vi "DiffDriveTrainSim_ToughBoxMiniGearRatio.vi"(11 "ToughBoxMiniGear":T1) -> (3 "GearRatio":dbl)   [LabVIEW 2019, in "Trajectory_Library.lvlib"]
doc: "Convience function to allow user to select kit bot gear ratio from an enum selector and return the ratio value\n\nInput:\n - StandardGearRatios -- Enumerated gear ratio selector\n\nOutput:\n - GearRatio -- Gear ratio value."
uses:
  Trajectory_Library.lvlib
  Enum/DIFF_DRIVE_ToughBoxMini_GearChoice_ENUM.ctl
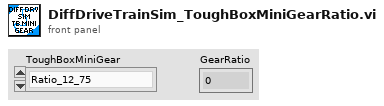
[diagram p1: front panel]
types:
  T1 = typedef "Trajectory_Library.lvlib/DIFF_DRIVE_ToughBoxMini_GearChoice_ENUM.ctl" = enum16{"Ratio_12_75", "Ratio_10_71", "Ratio_8_45", "Ratio_7_31", "Ratio_5_95"}
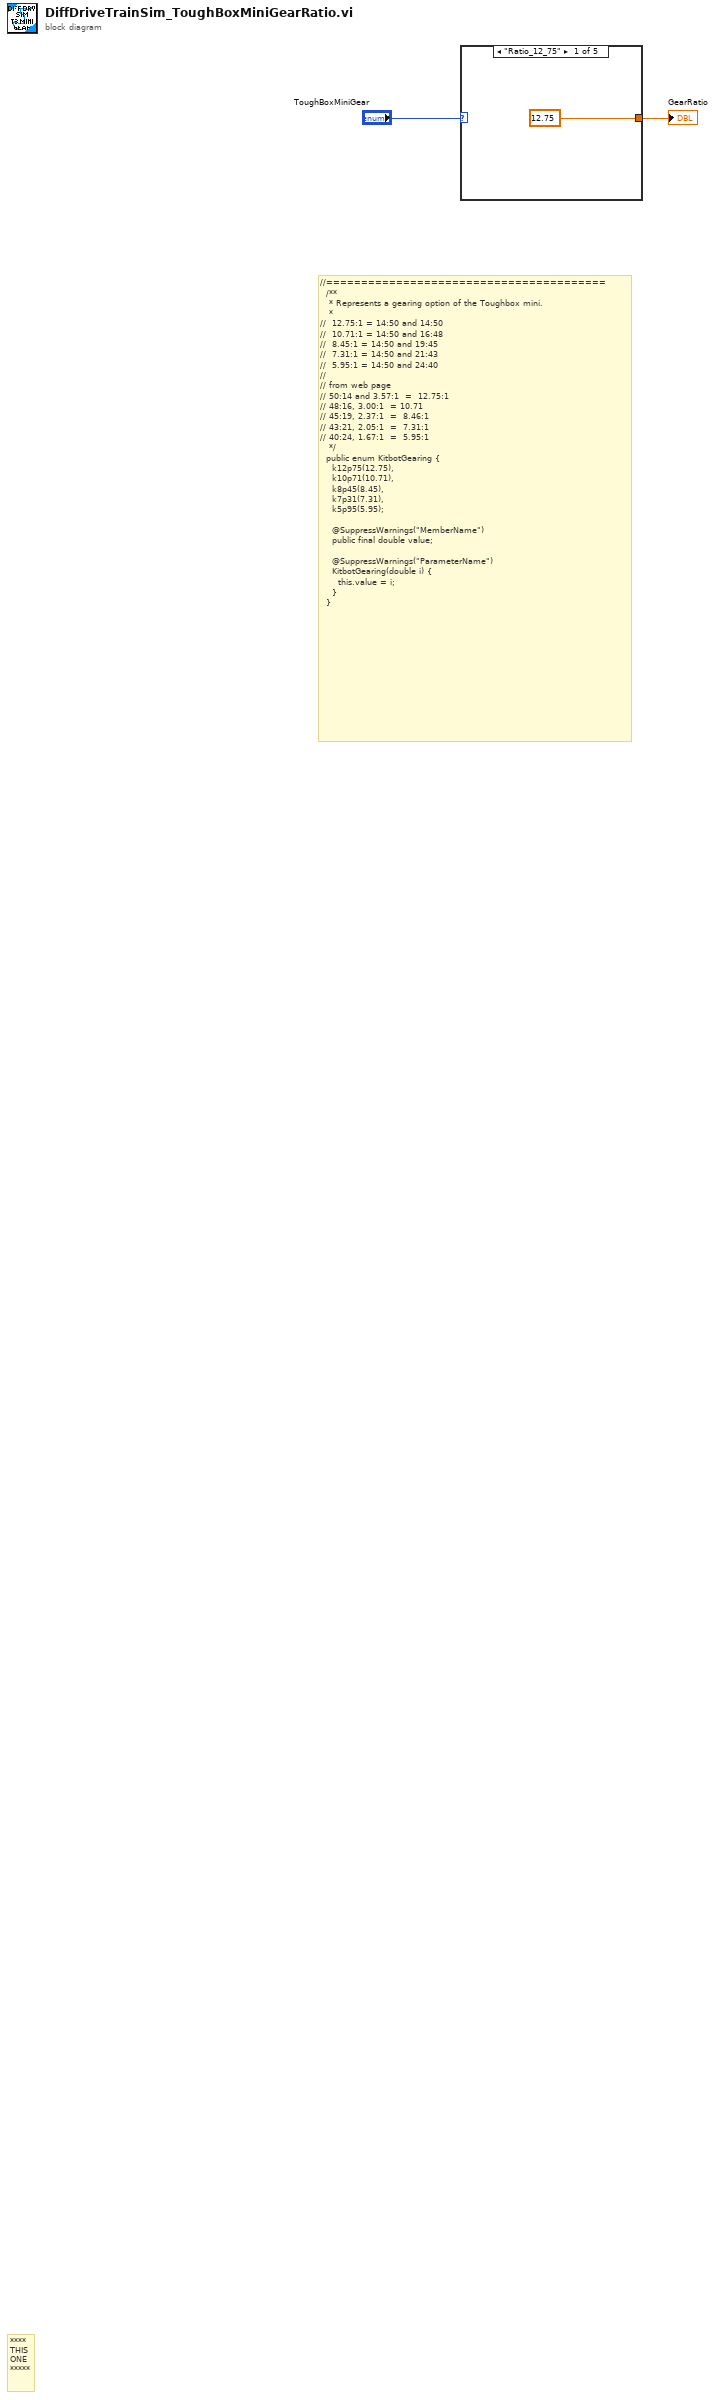
[diagram p0: block diagram]
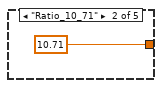
[diagram p2: hidden frame]
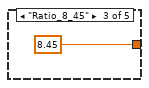
[diagram p3: hidden frame]
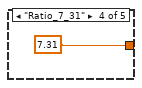
[diagram p4: hidden frame]
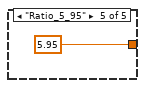
[diagram p5: hidden frame]
diagram:
  # "//========================================\n  /**\n   * Represents a gearing option of the Toughbox mini. \n   *\n//\t\t12.75:1 = 14:50 and 14:50 \n//\t\t10.71:1 = 14:50 and 16:48 \n//\t\t8.45:1 = 14:50 and 19:45\n//\t\t7.31:1 = 14:50 and 21:43\n//\t\t5.95:1 = 14:50 and 24:40\n//\n//\tfrom web page\n//\t50:14 and 3.57:1  =  12.75:1\n//\t48:16, 3.00:1  = 10.71\n//\t45:19, 2.37:1  =  8.46:1\n//\t43:21, 2.05:1  =  7.31:1\n//\t40:24, 1.67:1  =  5.95:1\n   */\n  public enum KitbotGearing {\n    k12p75(12.75),\n    k10p71(10.71),\n    k8p45(8.45),\n    k7p31(7.31),\n    k5p95(5.95);\n\n    @SuppressWarnings(\"MemberName\")\n    public final double value;\n\n    @SuppressWarnings(\"ParameterName\")\n    KitbotGearing(double i) {\n      this.value = i;\n    }\n  }"
  # "****\nTHIS\nONE\n*****"
  n1 = case shown="\"Ratio_12_75\"" "ToughBoxMiniGear" {
    tunnel: [12.75 10.71 8.45 7.31 5.95] -> w1
    frame "Ratio_12_75" {
    }
    frame "Ratio_10_71" {
    }
    frame "Ratio_8_45" {
    }
    frame "Ratio_7_31" {
    }
    frame "Ratio_5_95" {
    }
  }
  "GearRatio" <- w1
